vi "GD_GWID9_B.vi"(8 "error in (no error)":errorcluster, 11 "DBlink":string="Driver={ODBC Driver 17 for SQL Server};Server=localhost\\SQLEXPRESS;Database=ZDX201;UID=labview;PWD=Dsa@54137926") -> (0 "error out":errorcluster, 2 "glue_id":i32=16)   [LabVIEW 2019]
uses:
  <vilib>/addons/database/Connection.llb/DB Tools Open Connec (String).vi
  <vilib>/addons/database/Connection.llb/Conn Execute.vi
  <vilib>/addons/database/Recordset.llb/Rec Fetch Recordset Data (R).vi
  <vilib>/addons/database/Recordset.llb/Rec Destroy - Connection.vi
  <vilib>/addons/database/_DB Variant To Data/Database Variant To Data.xnode
  <vilib>/addons/database/NI_Database_API.lvlib
panel:
  out "Command 1":string="SELECT TOP (1) [id]      \n FROM [ZDX201].[dbo].[glue_data]\n where glue_workspace_id=9 and time_spout is not null\norder by id desc "
  out "Command 2":string="WHERE [id]=16"
  in  "columns":string[](array[string])=["glue_workspace_id", "update_time"]
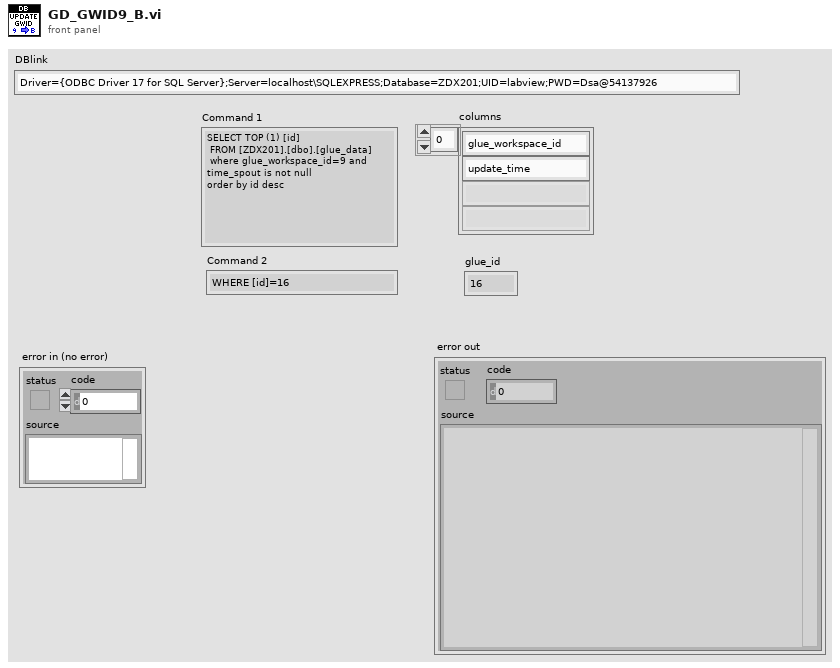
[diagram p1: front panel]
types:
  T1 = cluster{"Next GWID":i32, "update_time":timestamp}
  T2 = typedef "NI_Database_API.lvlib/Conn ObjectReference.ctl" = refnum<k1>
  T3 = typedef "NI_Database_API.lvlib/Rec ObjectReference.ctl" = refnum<k1>
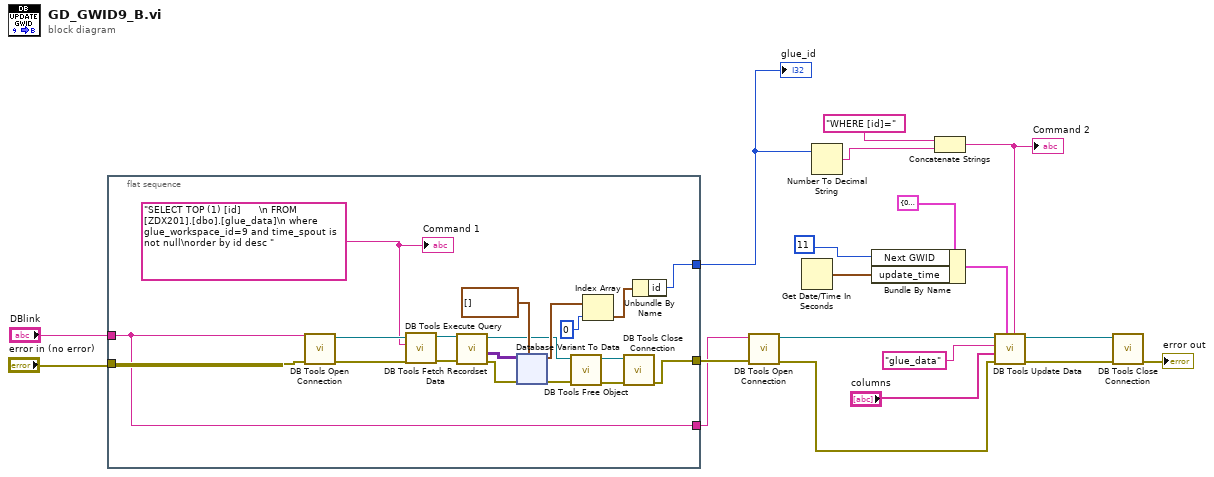
[diagram p0: block diagram]
diagram:
  n1 = flat-sequence {
    tunnel: "DBlink" -> [w24]
    tunnel: "error in (no error)" -> [w38]
    tunnel: [w25] -> w5
    tunnel: [w24] -> w4
    tunnel: [w21] -> w3
    frame #0 {
      w20 = "SELECT TOP (1) [id]      \n FROM [ZDX201].[dbo].[glue_data]\n where glue_workspace_id=9 and time_spout is not null\norder by id desc " ("SQL query")
      n2 = call-poly <vilib>:"DB Tools Open Connection.vi"("error in (no error)"=w38, "connection information"=w24) -> ("error out"=w37:errorcluster, "connection reference"=w36:T2)  [unwired: 6 in]
      n3 = call-poly <vilib>:"DB Tools Execute Query.vi"("error in (no error)"=w37, "SQL query"=w20, "connection reference"=w36) -> ("error out"=w35:errorcluster, "recordset reference"=w34:T3)  [unwired: 5 in]
      n4 = call-poly <vilib>:"DB Tools Fetch Recordset Data.vi"("error in (no error)"=w35, "recordset reference"=w34) -> ("error out"=w33:errorcluster, "recordset data"=w23:variant[][], "recordset reference out"=w26:T3)  [unwired: 3 in]
      n5 = xnode "Database Variant To Data"("database variant"=w23, "error in (no error)"=w33, "type"=cluster{"id":i32}[] [] ("initialized array")) -> ("data"=w31:cluster{"id":i32}[], "error out"=w27:errorcluster)
      n6 = call-poly <vilib>:"DB Tools Free Object.vi"("error in (no error)"=w27, "recordset reference"=w26) -> ("error out"=w28:errorcluster, "connection reference"=w29:T2)  [unwired: 8 in]
      n7 = Index Array(array=w31, index=0) -> (element=w22:cluster{"id":i32})
      n8 = call <vilib>:"DB Tools Close Connection.vi"("error in (no error)"=w28, "connection reference"=w29) -> ("error out"=w25:errorcluster)  [unwired: 5 in]
      n9 = Unbundle By Name(w22) -> ("id"=w21:i32)
      "Command 1" <- w20
    }
  }
  n10 = call-poly <vilib>:"DB Tools Open Connection.vi"("error in (no error)"=w5, "connection information"=w4) -> ("error out"=w18:errorcluster, "connection reference"=w8:T2)  [unwired: 6 in]
  n11 = Get Date/Time In Seconds() -> (seconds since 1Jan1904=w1:timestamp)
  n12 = Number To Decimal String(number=w3) -> (decimal integer string=w9:string)  [unwired: 1 in]
  n13 = Bundle By Name(cluster=T1 {"Next GWID"=0, "update_time"=timestamp(0 s since 1904-01-01)}, "Next GWID"=11, "update_time"=w1) -> (w10:T1)
  n14 = Concatenate Strings("WHERE [id]=", w9) -> (w12:string)
  "Command 2" <- w12
  n15 = call <vilib>:"DB Tools Update Data.vi"("condition"=w12, "data"=w10, "error in (no error)"=w18, "columns"="columns", "table"="glue_data", "connection reference"=w8) -> ("error out"=w19:errorcluster, "connection reference out"=w17:T2)  [unwired: 4 in]
  n16 = call <vilib>:"DB Tools Close Connection.vi"("error in (no error)"=w19, "connection reference"=w17) -> ("error out"=→"error out":errorcluster)  [unwired: 5 in]
  "glue_id" <- w3
